vi "GetArea.vi"(11 "Rectangle In":refnum<class "Rectangle.lvclass">) -> (2 "Area":dbl, 3 "Rectangle Out":refnum<class "Rectangle.lvclass">)   [LabVIEW 2018, in "Rectangle.lvclass"]
uses:
  Rectangle.lvclass
  Rectangle.lvclass/Rectangle.ctl
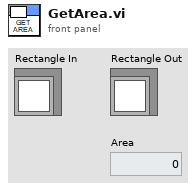
[diagram p1: front panel]
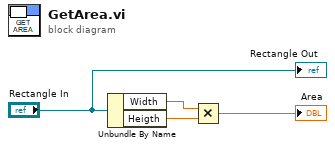
[diagram p0: block diagram]
diagram:
  n1 = Unbundle By Name("Rectangle In") -> ("Width"=w2:dbl, "Heigth"=w3:dbl)
  n2 = Multiply(x=w2, y=w3) -> (x*y=→"Area":dbl)
  "Rectangle Out" <- "Rectangle In"
